vi "Get 1D String.vi"(5 "format string (%s)":string="%s", 7 "key description":string, 8 "sections":string[](array[string]), 9 "string":string[](array[string]), 11 "info data":string) -> (0 "sections out":string[](array[string]), 1 "found?":bool, 2 "value":string[](array[string]), 3 "info data out":string)   [LabVIEW 2013, in "infolib.lvlib"]
doc: "Reads horizontal or vertical vector of strings. If section is entered it searches the key in the section(s)."
uses:
  infolib.lvlib
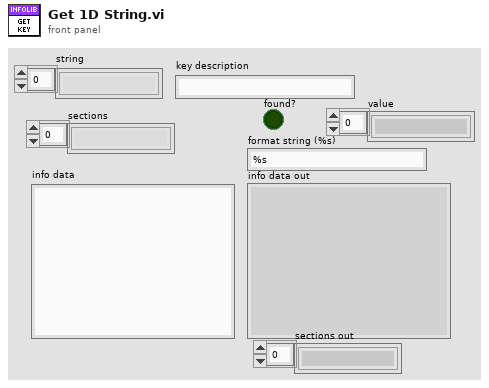
[diagram p1: front panel]
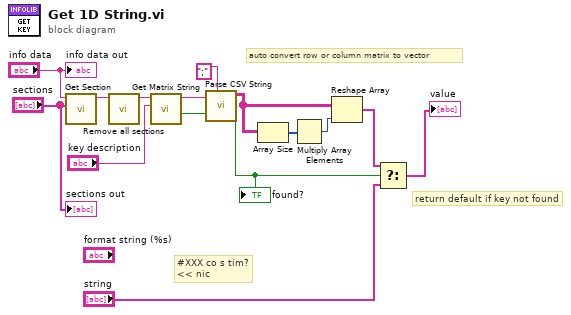
[diagram p0: block diagram]
diagram:
  # "return default if key not found"
  # "#XXX co s tim?\n<< nic"
  # "auto convert row or column matrix to vector"
  n1 = call "Get Section.vi"("sections"="sections", "info data"="info data") -> ("section part"=w14:string)  [unwired: 8 in, 1 out]
  n2 = call "Remove all sections.vi"("info data"=w14) -> ("info data out"=w11:string)  [unwired: 10 in]
  n3 = call "Get Matrix String.vi"("matrix key"="key description", "info data"=w11) -> ("exist"=w4:bool, "matrix part"=w7:string)  [unwired: 8 in]
  "found?" <- w4
  n4 = call "Parse CSV String.vi"("delimiter (,)"=";" ("delimiter (Tab)"), "CSV string"=w7) -> ("2-D array"=w5:string[][])  [unwired: 8 in, 1 out]
  n5 = Array Size(array=w5) -> (size(s)=w9:i32[])
  n6 = Multiply Array Elements(1:w9) -> (0:w8:i32)
  n7 = Reshape Array(w5, w8) -> (w3:string[])
  n8 = Select(t=w3, s=w4, f="string") -> (s? t:f=→"value":string[])
  "info data out" <- "info data"
  "sections out" <- "sections"
